vi "Read StimulationPath.vi"(8 "error in (no error)":errorcluster, 11 "MatlabExperiment in":refnum<class "MatlabExperiment.lvclass">) -> (0 "error out":errorcluster, 2 "StimulationPath":path, 3 "MatlabExperiment out":refnum<class "MatlabExperiment.lvclass">)   [LabVIEW 2010, in "MatlabExperiment.lvclass"]
uses:
  MatlabExperiment.lvclass
  MatlabExperiment.lvclass/MatlabExperiment.ctl
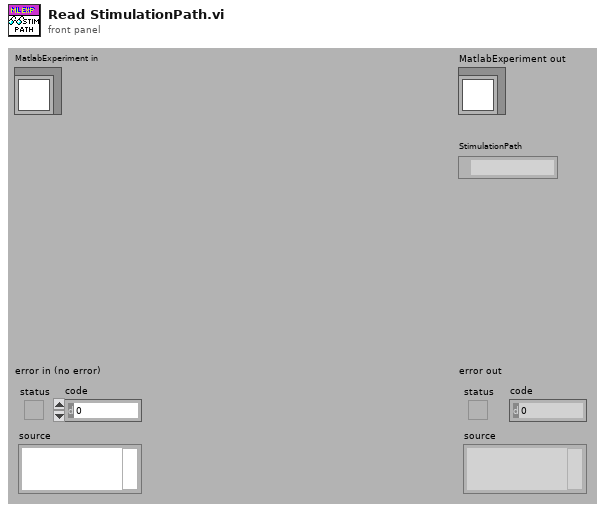
[diagram p1: front panel]
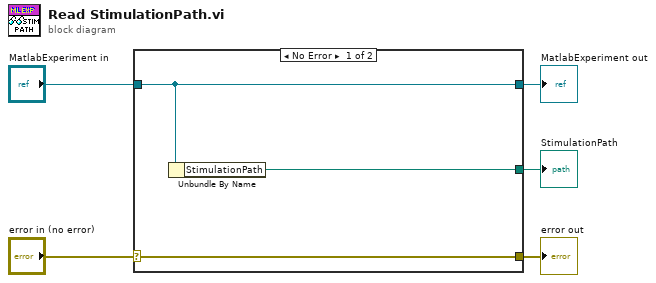
[diagram p0: block diagram]
diagram:
  n1 = case shown="No Error" "error in (no error)" {
    selector: "error in (no error)" -> [w8 w9]
    tunnel: [w8 w9] -> w4
    tunnel: [w7 w10] -> w2
    tunnel: "MatlabExperiment in" -> [w7 w10]
    tunnel: [w6 _] -> w1
    frame No Error {
      n2 = Unbundle By Name(w7) -> ("StimulationPath"=w6:path)
    }
    frame Error {
    }
  }
  "error out" <- w4
  "MatlabExperiment out" <- w2
  "StimulationPath" <- w1
